vi "POV Conditioning.vi"(11 "POV":i16) -> (3 "Output [-1-4]":i16)   [LabVIEW 2018, in "Joysticks.lvlib" / "Joysticks.lvclass"]
doc: "This VI conditions the D-Pad from a 360 degree output to quadrant only."
uses:
  Joysticks.lvclass
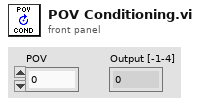
[diagram p1: front panel]
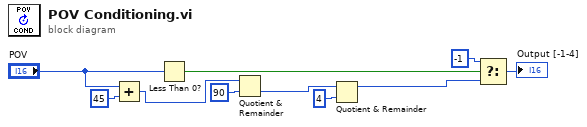
[diagram p0: block diagram]
diagram:
  n1 = Add(x="POV", y=i16 45) -> (x+y=w7:i16)
  n2 = Less Than 0?(x="POV") -> (x < 0?=w4:bool)
  n3 = Quotient & Remainder(x=w7, y=i16 90) -> (floor(x/y)=w9:i16)  [unwired: 1 out]
  n4 = Quotient & Remainder(x=w9, y=i16 4) -> (x-y*floor(x/y)=w2:i16)  [unwired: 1 out]
  n5 = Select(t=i16 -1, s=w4, f=w2) -> (s? t:f=→"Output [-1-4]":i16)
